vi "Apply.vi"(8 "error in":errorcluster, 11 "Thermometer DAQmx RTD Cont CFG in":refnum<class "Thermometer DAQmx TC Cont CFG Simulated.lvclass">) -> (0 "error out":errorcluster, 3 "Thermometer DAQmx RTD Cont CFG out":refnum<class "Thermometer DAQmx TC Cont CFG Simulated.lvclass">)   [LabVIEW 2024, in "DAQmx Simulated CFGs.lvlib" / "Thermometer DAQmx TC Cont CFG Simulated.lvclass"]
uses:
  Thermometer DAQmx TC Cont CFG Simulated.lvclass
  Thermometer DAQmx TC Cont CFG Simulated.lvclass/Thermometer DAQmx TC Cont CFG Simulated.ctl
  Thermometer DAQmx TC Cont CFG/Thermometer DAQmx TC Cont CFG.lvclass
  Configurations/CFG Base/CFG Base.lvclass
  D:/git/HAL/HAL/Devices/DAQmx/Thermo/Thermometer DAQmx TC Cont CFG/Thermometer DAQmx TC Cont CFG.lvclass
  D:/git/HAL/HAL/Devices/DAQmx/DAQmx Base CFG/DAQmx Base CFG.lvclass
  D:/git/HAL/HAL/Configurations/CFG JSON/CFG JSON.lvclass
  D:/git/HAL/HAL/Configurations/CFG Base/CFG Base.lvclass
  D:/git/HAL/HAL/Devices/DAQmx/Thermo/Thermometer Simulated CFGs/TC Cont CFG/Thermometer DAQmx TC Cont CFG Simulated.lvclass
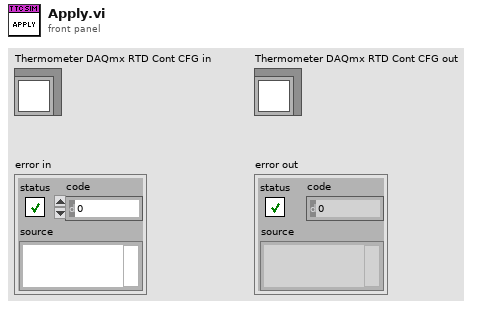
[diagram p1: front panel]
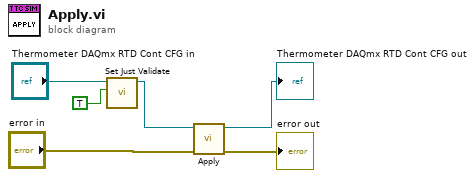
[diagram p0: block diagram]
diagram:
  n1 = call "Set Just Validate.vi"("Just Validate"=TRUE, "CFG Base in"="Thermometer DAQmx RTD Cont CFG in") -> ("CFG Base out"=w1:refnum<class "Thermometer DAQmx TC Cont CFG Simulated.lvclass">)  [unwired: 9 in]
  n2 = call-parent "Apply.vi"("error in"="error in", "Thermometer DAQmx RTD Cont CFG in"=w1) -> ("error out"=→"error out":errorcluster, "Thermometer DAQmx RTD Cont CFG out"=→"Thermometer DAQmx RTD Cont CFG out":refnum<class "Thermometer DAQmx TC Cont CFG Simulated.lvclass">)  [unwired: 8 in]
